vi "MT_DATA_TRANS(SubVI).vi"(11 "MT_DATA":sgl[](array[numeric])) -> (3 "MT_DATA_T":dbl[](array[numeric]))   [LabVIEW 2011]
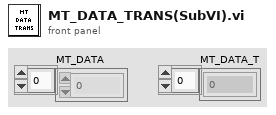
[diagram p1: front panel]
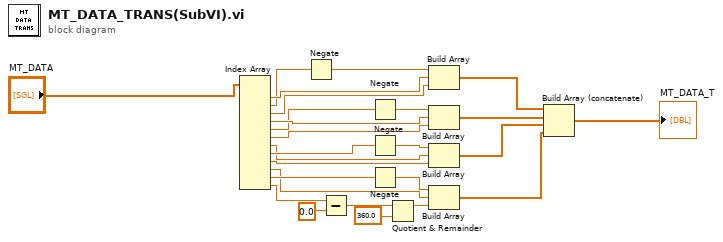
[diagram p0: block diagram]
diagram:
  n1 = Index Array(array="MT_DATA") -> (element #1=w4:sgl, element #2=w2:sgl, element #3=w5:sgl, element #4=w9:sgl, element #5=w8:sgl, element #6=w11:sgl, element #7=w12:sgl, element #8=w13:sgl, element #9=w14:sgl, element #10=w16:sgl, element #11=w17:sgl, element #12=w18:sgl)  [unwired: 12 in]
  n2 = Negate(x=w2) -> (-x=w3:sgl)
  n3 = Subtract(x=w18, y=sgl 0.0) -> (x-y=w20:sgl)
  n4 = Negate(x=w8) -> (-x=w7:sgl)
  n5 = Negate(x=w13) -> (-x=w6:sgl)
  n6 = Negate(x=w17) -> (-x=w15:sgl)
  n7 = Quotient & Remainder(x=w20, y=360.0) -> (x-y*floor(x/y)=w21:dbl)  [unwired: 1 out]
  n8 = Build Array(w3, w4, w5) -> (w22:sgl[])
  n9 = Build Array(w7, w9, w11) -> (w23:sgl[])
  n10 = Build Array(w6, w12, w14) -> (w24:sgl[])
  n11 = Build Array(w15, w16, w21) -> (w25:dbl[])
  n12 = Build Array (concatenate)(w22, w23, w24, w25) -> (→"MT_DATA_T":dbl[])
